vi "Roller Motor Logic Test.vi"() -> ()   [LabVIEW 2013]
panel:
  out "Solenoid out":bool
  out "Roller Output":dbl
  in  "Roller Speed":dbl
  in  "Command":enum16{"Stop", "Forward", "Reverse"}(ring)
  in  "stop":bool
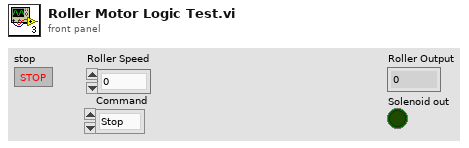
[diagram p1: front panel]
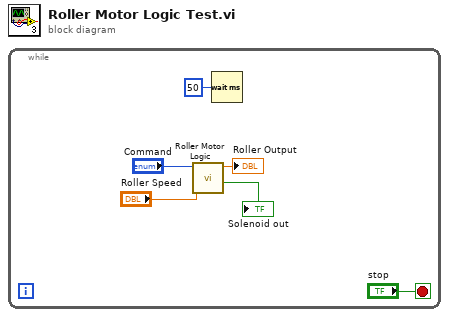
[diagram p0: block diagram]
diagram:
  n1 = while {
    stop <- "stop" stop-if-true
    n2 = call "Roller Motor Logic.vi"("Roller Speed"="Roller Speed", "Command"="Command") -> ("Solenoid out"=→"Solenoid out":bool, "Roller Output"=→"Roller Output":dbl)  [unwired: 8 in]
    n3 = Wait (ms)(milliseconds to wait=u32 50) -> ()  [unwired: 1 out]
  }
